vi "LEP_RV_OnBuild.vi"(8 "error in (no error)":errorcluster) -> (0 "error out":errorcluster)   [LabVIEW 2011]
doc: "Download and execute built VxWorks downloadable module and attach the LabVIEW Embedded debuger."
uses:
  LEP_RV_Commands.ctl
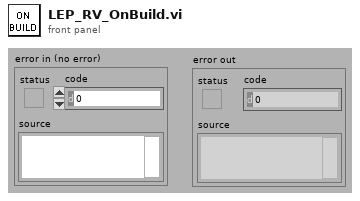
[diagram p1: front panel]
types:
  T1 = typedef "LEP_RV_Commands.ctl" = enum16{"Build", "Rebuild", "Run", "Debug", "Profile"}
  T2 = typedef "LEP_RV_Config.ctl" = cluster{"Enable debugging":bool, "Debug Options":u16, "Use stack variables":bool, "Generate serial only":bool, "Generate guard code":bool, "Generate Integer Only":bool, "Generate C Function Calls":bool, "ExpressionFolding":bool, "Constant Allocation":u16, "Constant Deallocation":u16, "Build Specification ID":string, "Preprocessor symbols (define)":string, "Compiler Flags":string, "Linker Flags":string, "Mode":u16, "Optimization":u16, "Optimize for time":bool, "Enable cross-module optimization":bool, "Include paths":path[], "Optimize heap size":bool, "Use MicroLib":bool, "Debug Mode":u16, "Enable profile information":bool, "Host name":string, "Use DHCP":bool, "IP address":string, "Subnet mask":string, "Gateway":string, "Primary DNS":string, "Secondary DNS":string, "MAC in target memory":bool, "MAC address":string, "Console output":u16, "Target serial port":u16}
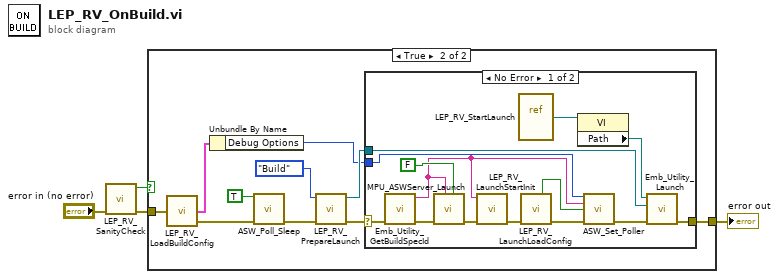
[diagram p0: block diagram]
diagram:
  n1 = call "LEP_RV_SanityCheck.vi"("error in (no error)"="error in (no error)") -> ("error out"=w2:errorcluster, "ok"=w1:bool)  [unwired: 1 in, 8 out]
  n2 = case shown="True" w1 {
    tunnel: [w5 w7] -> w3
    tunnel: w2 -> [w5 w6]
    frame False {
    }
    frame True {
      n3 = call "LEP_RV_LoadBuildConfig.vi"("error in (no error)"=w6) -> ("Config"=w12:T2, "error out"=w8:errorcluster)  [unwired: 1 out]
      n4 = Unbundle By Name(w12) -> ("Debug Options"=w11:u16)
      n5 = call <vilib>:"ASW_Poll_Sleep.vi"("Sleep"=TRUE, "error in (no error)"=w8) -> ("error out"=w10:errorcluster)  [unwired: 13 in]
      n6 = call "LEP_RV_PrepareLaunch.vi"("error in (no error)"=w10, "Commands"=LEP_RV_Commands."Build") -> ("error out"=w14:errorcluster, "output cluster"=w13:refnum<vi>)  [unwired: 7 in, 1 out]
      n7 = case shown="No Error" w14 {
        selector: w14 -> [w25 w30]
        tunnel: [w29 w30] -> w7
        tunnel: w13 -> [w24 _]
        tunnel: w11 -> [w22 _]
        frame No Error {
          n8 = call <vilib>:"Emb_Utility_GetBuildSpecId.vi"("error in (no error)"=w25) -> ("error out"=w26:errorcluster, "buildSpec ID"=w20:string)  [unwired: 7 out]
          n9 = call <vilib>:"MPU_ASWServer_Launch.vi"("initialize (T)"=FALSE, "buildSpec ID"=w20, "error in"=w26) -> ("error out"=w19:errorcluster)  [unwired: 8 out]
          n10 = call "LEP_RV_LaunchStartInit.vi"("error in (no error)"=w19, "buildSpec ID"=w20) -> ("error out"=w18:errorcluster)  [unwired: 9 in]
          n11 = vi-ref "LEP_RV_StartLaunch.vi"() -> (w28:refnum<vi>)
          n12 = call "LEP_RV_LaunchLoadConfig.vi"("error in (no error)"=w18) -> ("Connect to a network compile server"=w16:bool, "error out"=w17:errorcluster)  [unwired: 7 in, 6 out]
          n13 = property class="VI"(reference=w28) -> ("Path"=w27:path)  [unwired: 1 in, 2 out]
          n14 = call <vilib>:"ASW_Set_Poller.vi"("Debug Options"=w22, "buildSpec ID"=w20, "Connect to a network compile server"=w16, "error in (no error)"=w17) -> ("error out"=w21:errorcluster)  [unwired: 11 in]
          n15 = call <vilib>:"Emb_Utility_Launch.vi"("error in"=w21, "parameter cluster"=w24, "vi path"=w27) -> ("error out"=w29:errorcluster)  [unwired: 6 out]
        }
        frame Error {
        }
      }
    }
  }
  "error out" <- w3
